vi "checkRegCmdRule.vi"(8 "error in (no error)":errorcluster, 10 "tcpPacket":string, 11 "tcpServerCmd in":refnum<class "TcpServerCmd.lvclass">) -> (0 "error out":errorcluster, 1 "regCmd?":bool, 2 "tcpPacket":string, 3 "tcpServerCmd out":refnum<class "TcpServerCmd.lvclass">)   [LabVIEW 2018, in "TcpServerCmd.lvclass"]
doc: "Check if command received is in the registered commands list. If is ok, it sends the commands as an user event to the User."
uses:
  TcpServerCmd.lvclass
  TcpServerCmd.lvclass/TcpServerCmd.ctl
  <vilib>/regexp/Match Regular Expression.xnode
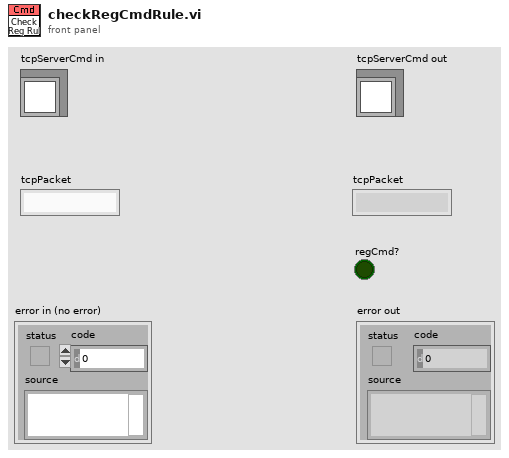
[diagram p1: front panel]
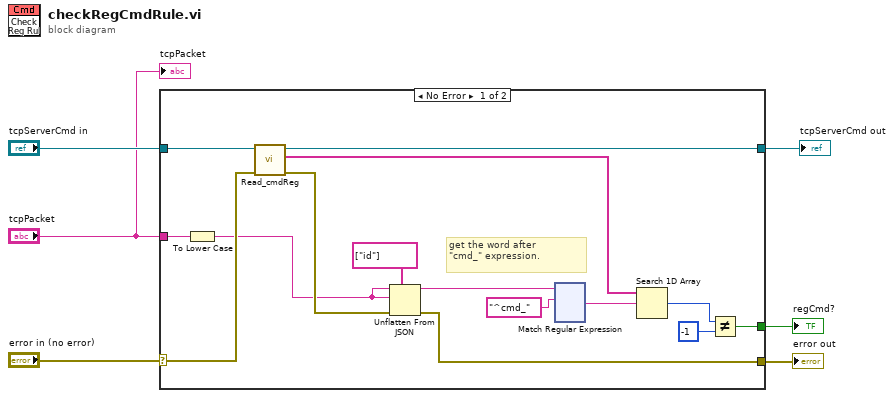
[diagram p0: block diagram]
diagram:
  n1 = case shown="No Error" "error in (no error)" {
    selector: "error in (no error)" -> [w13 w137]
    tunnel: [w17 w137] -> w3
    tunnel: [w14 w136] -> w4
    tunnel: "tcpServerCmd in" -> [w16 w136]
    tunnel: [w19 _] -> w2
    tunnel: "tcpPacket" -> [w8 _]
    frame No Error {
      # "get the word after\n\"cmd_\" expression."
      n2 = To Lower Case(string=w8) -> (all lower case string=w7:string)
      n3 = call "Read_cmdReg.vi"("error in (no error)"=w13, "TcpServerCmd in"=w16) -> ("error out"=w12:errorcluster, "cmdReg"=w15:string[], "TcpServerCmd out"=w14:refnum<class "TcpServerCmd.lvclass">)  [unwired: 7 in]
      n4 = Unflatten From JSON(path=string[] ["id"] ("tcp packet"), JSON string=w7, type and defaults=w7, error in (no error)=w12) -> (value=w11:string, error out=w17:errorcluster)  [unwired: 3 in]
      n5 = xnode "Match Regular Expression"("input string"=w11, "regular expression"="^cmd_") -> ("after match"=w9:string)  [unwired: 4 in, 4 out]
      n6 = Search 1D Array(1D array=w15, element=w9) -> (index of element=w21:i32)  [unwired: 1 in]
      n7 = Not Equal?(x=w21, y=-1) -> (x != y?=w19:bool)
    }
    frame Error {
    }
  }
  "error out" <- w3
  "tcpServerCmd out" <- w4
  "regCmd?" <- w2
  "tcpPacket" <- "tcpPacket"
